vi "Read Data.vi"(8 "error in (no error)":errorcluster, 11 "AI Driver in":refnum<class "AI Driver.lvclass">) -> (0 "error out":errorcluster, 2 "Daq Data":T1, 3 "AI Driver out":refnum<class "AI Driver.lvclass">)   [LabVIEW 2022 SP3, in "AI Driver.lvclass"]
uses:
  AI Driver.lvclass
  DAQ Data/AIDAQ Data.ctl
  DAQ Data/AI Daq Data.lvlib
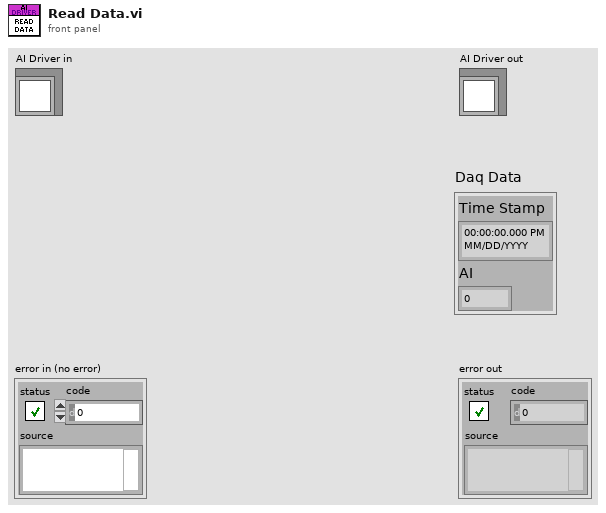
[diagram p1: front panel]
types:
  T1 = typedef "AI Daq Data.lvlib/AIDAQ Data.ctl" = cluster{"Time Stamp":timestamp, "AI":dbl}
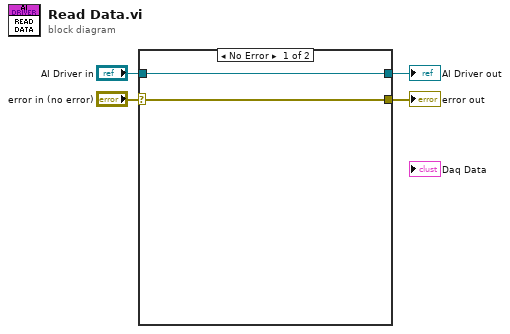
[diagram p0: block diagram]
diagram:
  n1 = case shown="No Error" "error in (no error)" {
    selector: "error in (no error)" -> [w5 w8]
    tunnel: [w5 w8] -> w3
    tunnel: [w6 w7] -> w1
    tunnel: "AI Driver in" -> [w6 w7]
    frame No Error {
    }
    frame Error {
    }
  }
  "error out" <- w3
  "AI Driver out" <- w1
